vi "Overlay Crosshairs.vi"(0 "Image In":T1=refnum, 1 "Coordinates":cluster{"X":dbl, "Y":dbl}, 2 "Crosshair Length (px)":dbl, 3 "Crosshair Thickness":i32, 4 "Color":u32(colorbox)=15663156) -> (6 "Image Out":T1)   [LabVIEW 2015]
uses:
  <vilib>/vision/Image Controls.llb/IMAQ Image.ctl
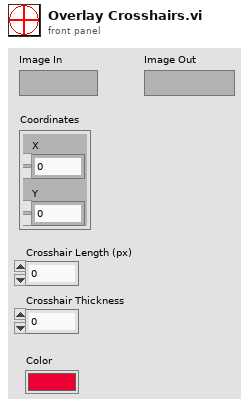
[diagram p1: front panel]
types:
  T1 = typedef "IMAQ Image.ctl" = refnum<image>
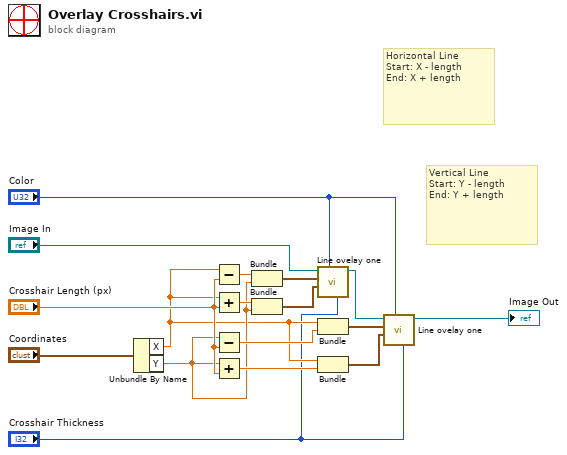
[diagram p0: block diagram]
diagram:
  # "Vertical Line\nStart: Y - length\nEnd: Y + length"
  # "Horizontal Line\nStart: X - length\nEnd: X + length"
  n1 = Unbundle By Name("Coordinates") -> ("X"=w2:dbl, "Y"=w3:dbl)
  n2 = Subtract(x=w2, y="Crosshair Length (px)") -> (x-y=w15:dbl)
  n3 = Add(x=w2, y="Crosshair Length (px)") -> (x+y=w12:dbl)
  n4 = Subtract(x=w3, y="Crosshair Length (px)") -> (x-y=w6:dbl)
  n5 = Add(x=w3, y="Crosshair Length (px)") -> (x+y=w4:dbl)
  n6 = Bundle(w15, "Y"=w3) -> (w14:cluster{dbl, "Y":dbl})  [unwired: 1 in]
  n7 = Bundle(w12, "Y"=w3) -> (w13:cluster{dbl, "Y":dbl})  [unwired: 1 in]
  n8 = call "Line ovelay one.vi"("Thickness"="Crosshair Thickness", "Color"="Color", "End Point"=w13, "Start Point"=w14, "Image"="Image In") -> ("Image Out"=w10:T1)  [unwired: 5 in, 1 out]
  n9 = Bundle("X"=w2, w6) -> (w9:cluster{"X":dbl, dbl})  [unwired: 1 in]
  n10 = Bundle("X"=w2, w4) -> (w8:cluster{"X":dbl, dbl})  [unwired: 1 in]
  n11 = call "Line ovelay one.vi"("Thickness"="Crosshair Thickness", "Color"="Color", "End Point"=w8, "Start Point"=w9, "Image"=w10) -> ("Image Out"=→"Image Out":T1)  [unwired: 5 in, 1 out]
